vi "getClientStatus.vi"(8 "error in (no error)":errorcluster, 11 "TcpServer in":refnum<class "TcpServer.lvclass">) -> (0 "error out":errorcluster, 3 "TcpServer out":refnum<class "TcpServer.lvclass">)   [LabVIEW 2018, in "TcpServer.lvclass"]
doc: "Get the notification from TCP Server that TCP Client connects or disconnects and then send an user event to the Component."
uses:
  TcpServer.lvclass
  TcpServerBase/typedef/connStatusCluster.ctl
  TcpServerCmd/TcpServerCmd.lvclass
  TcpServerBase/TcpServerBase.lvclass
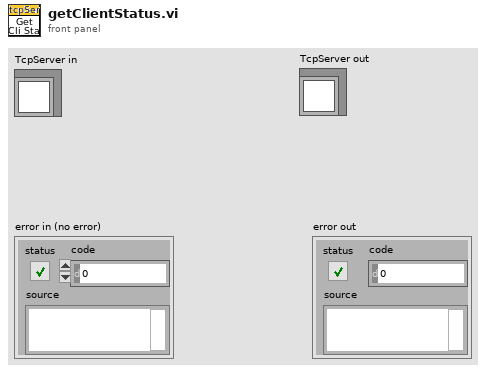
[diagram p1: front panel]
types:
  T1 = typedef "TcpServerBase.lvclass/connStatusCluster.ctl" = cluster{"connStatus":bool, "message":string}
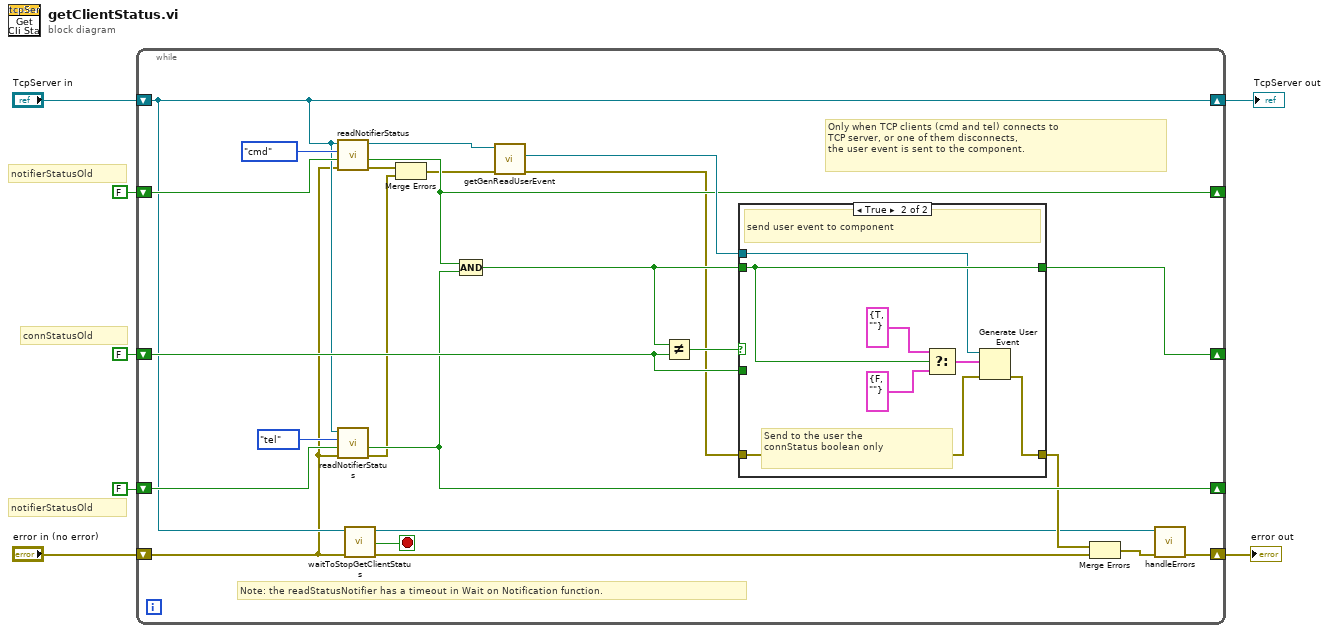
[diagram p0: block diagram]
diagram:
  # "notifierStatusOld"
  # "notifierStatusOld"
  # "connStatusOld"
  n1 = while {
    shift-right: [w20] -> w6
    shift-left: "TcpServer in" -> [w20]
    shift-right: [w22] -> _
    shift-left: FALSE ("connectionStatus") -> [w24]
    shift-right: [w21] -> _
    shift-left: FALSE ("connectionStatus") -> [w23]
    shift-right: [w29] -> _
    shift-left: FALSE ("connectionStatus") -> [w28]
    shift-right: [w9] -> w1
    shift-left: "error in (no error)" -> [w19]
    stop <- w16 stop-if-true
    # "Only when TCP clients (cmd and tel) connects to\nTCP server, or one of them disconnects,\nthe user event is sent to the component."
    # "Note: the readStatusNotifier has a timeout in Wait on Notification function."
    n2 = call "readNotifierStatus.vi"("error in (no error)"=w19, "notifierStatusOld"=w24, "serverSelection"=enum16{"cmd", "tel"}."cmd" ("server"), "TcpServer in"=w20) -> ("error out (no error)"=w14:errorcluster, "notifierStatusNew"=w22:bool, "TcpServer out"=w8:refnum<class "TcpServer.lvclass">)  [unwired: 5 in]
    n3 = call "readNotifierStatus.vi"("error in (no error)"=w19, "notifierStatusOld"=w23, "serverSelection"=enum16{"cmd", "tel"}."tel" ("server"), "TcpServer in"=w20) -> ("error out (no error)"=w13:errorcluster, "notifierStatusNew"=w21:bool)  [unwired: 5 in, 1 out]
    n4 = call "waitToStopGetClientStatus.vi"("error in (no error)"=w19, "tcpServer in"=w20) -> ("error out"=w18:errorcluster, "stop"=w16:bool, "tcpServer out"=w10:refnum<class "TcpServer.lvclass">)  [unwired: 7 in]
    n5 = Merge Errors(w14, w13) -> (w12:errorcluster)
    n6 = Compound Arithmetic op=AND(w22, w21) -> (w30:bool)
    n7 = call "getGenReadUserEvent.vi"("error in (no error)"=w12, "TcpServer in"=w8) -> ("error out"=w15:errorcluster, "GenRead"=w27:refnum<user-event>)  [unwired: 7 in, 1 out]
    n8 = Not Equal?(x=w30, y=w28) -> (x != y?=w31:bool)
    n9 = case shown="True" w31 {
      tunnel: w30 -> [_ w40]
      tunnel: [w33 w40] -> w29
      tunnel: w28 -> [w33 _]
      tunnel: w27 -> [_ w39]
      tunnel: [w32 w38] -> w17
      tunnel: w15 -> [w32 w37]
      frame False {
        # "do nothing"
      }
      frame True {
        # "Send to the user the\nconnStatus boolean only"
        # "send user event to component"
        n10 = Select(t=T1 {"connStatus"=TRUE, "message"=""}, s=w40, f=T1 {"connStatus"=FALSE, "message"=""} ("t")) -> (s? t:f=w36:T1)
        n11 = Generate User Event(user event=w39, event data cluster=w36, error in=w37) -> (error out=w38:errorcluster)  [unwired: 1 in, 1 out]
      }
    }
    n12 = Merge Errors(w17, w18) -> (w11:errorcluster)
    n13 = call "handleErrors.vi"("error in (no error)"=w11, "TcpServer in"=w10) -> ("error out"=w9:errorcluster)  [unwired: 8 in, 1 out]
  }
  "error out" <- w1
  "TcpServer out" <- w6
